vi "Serialize CRDS.vi"() -> ()   [LabVIEW 2012]
uses:
  CRDS/cCRDS/cCRDS.lvclass
  <userlib>/Serialization/Formatter/Formatter.lvclass
  <userlib>/Serialization/Formatter/Formatter.lvclass/Formatter.ctl
panel:
  out "error out":errorcluster
  out "JSON String":string
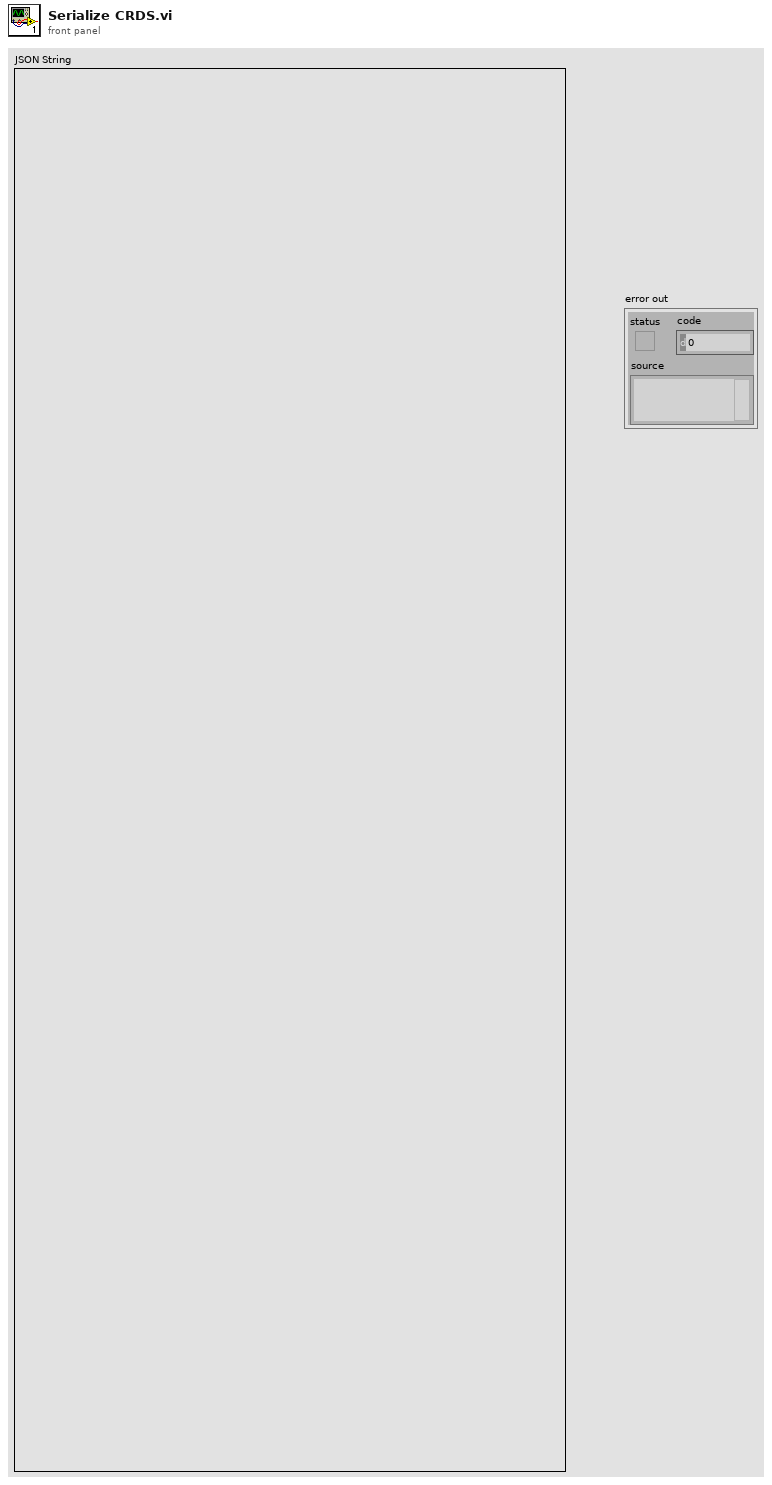
[diagram p1: front panel]
types:
  T1 = enum16{"No paths embedded", "One path with each object", "All paths with top object"}
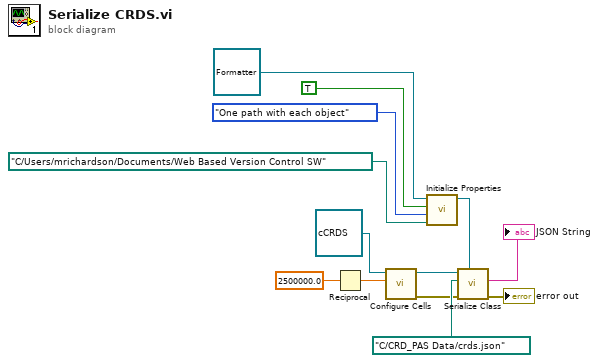
[diagram p0: block diagram]
diagram:
  n1 = Reciprocal(x=2500000.0) -> (1/x=w11:dbl)
  n2 = call "Configure Cells.vi"("dt"=w11, "cCRDS in"=refnum<class "cCRDS.lvclass"> refnum ("cCRDS")) -> ("error out"=w8:errorcluster, "cCRDS out"=w10:refnum<class "cCRDS.lvclass">)  [unwired: 8 in]
  n3 = call <userlib>:"Initialize Properties.vi"("Absolute Path For Dynamic Loading"=path "C:/Users/mrichardson/Documents/Web Based Version Control SW", "Path Embedding"=T1."One path with each object", "Include all fields?"=TRUE, "Formatter in (Default Formatter)"=refnum<class "Formatter.lvclass"> refnum) -> ("Formatter out"=w2:refnum<class "Formatter.lvclass">)  [unwired: 7 in]
  n4 = call-dynamic "Serialize Class.vi"("Formatter"=w2, "error in"=w8, "file path"=path "C:/CRD_PAS Data/crds.json", "Instrument in"=w10) -> ("error out"=→"error out":errorcluster, "JSON String"=→"JSON String":string)  [unwired: 5 in, 1 out]
